vi "New.vi"(8 "error in (no error)":errorcluster, 10 "Name":string, 11 "User Control in":refnum<class "Sequencer.lvclass">) -> (0 "error out":errorcluster, 3 "User Control out":refnum<class "Sequencer.lvclass">)   [LabVIEW 2024, in "Ramses Sequencer.lvlib" / "Sequencer.lvclass"]
uses:
  Sequencer.lvclass
  Sequence/Sequence.lvclass
  typedef/Sequencer State -- enum.ctl
  Program Files (x86)/Enterative/Ramses Framework/Ramses Framework.lvlibp/Service/Service.lvclass
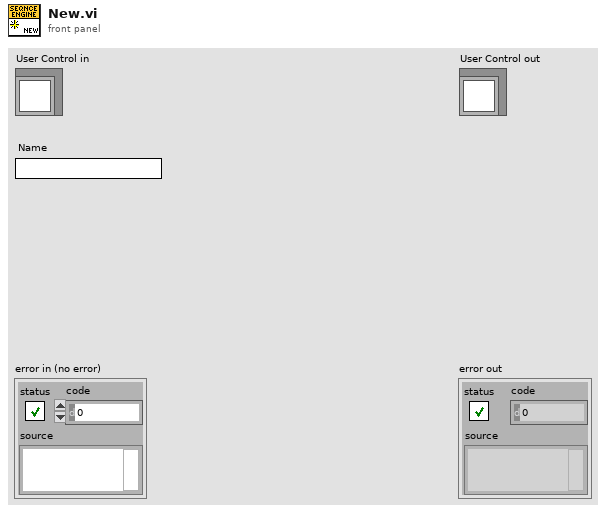
[diagram p1: front panel]
types:
  T1 = typedef "Ramses Sequencer.lvlib/Sequencer.lvclass/Sequencer State -- enum.ctl" = enum16{"Idle", "Running", "Paused", "Complete"}
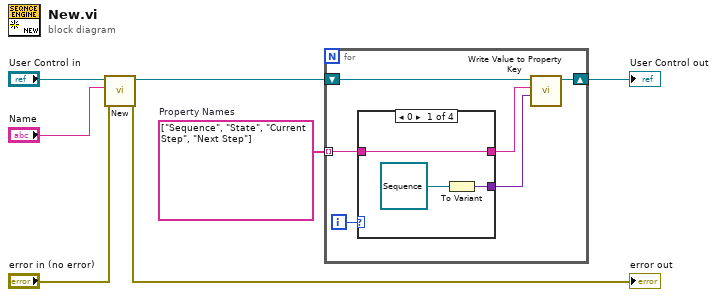
[diagram p0: block diagram]
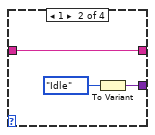
[diagram p2: hidden frame]
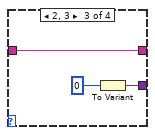
[diagram p3: hidden frame]
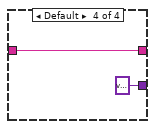
[diagram p4: hidden frame]
diagram:
  w2 = string[] ["Sequence", "State", "Current Step", "Next Step"]  # Property Names
  n1 = call-parent "New.vi"("error in (no error)"="error in (no error)", "Name"="Name", "Service in"="User Control in") -> ("error out"=→"error out":errorcluster, "Service out"=w5:refnum<class "Sequencer.lvclass">)  [unwired: 7 in]
  n2 = for {
    shift-right: [w10] -> w3
    shift-left: w5 -> [w11]
    tunnel: w2 -> [w12] mode=indexing
    i -> [w13]
    n3 = case shown="0" w13 {
      tunnel: [w16 w19 w22 variant ("Variant")] -> w8
      tunnel: w12 -> [w15 w18 w21 w24]
      tunnel: [w15 w18 w21 w24] -> w9
      frame 0 {
        n4 = To Variant(anything=refnum<class "Sequence.lvclass"> refnum ("RMS Sequencer.lvlib:Sequence.lvclass")) -> (Variant=w16:variant)
      }
      frame 1 {
        n5 = To Variant(anything=Sequencer_State_--_enum."Idle" ("Sequencer State")) -> (Variant=w19:variant)
      }
      frame 2, 3 {
        n6 = To Variant(anything=u32 0) -> (Variant=w22:variant)
      }
      frame Default {
      }
    }
    n7 = call "Write Value to Property Key.vi"("Value"=w8, "Key"=w9, "Service in"=w11) -> ("Service out"=w10:refnum<class "Sequencer.lvclass">)  [unwired: 7 in, 1 out]
  }
  "User Control out" <- w3
